vi "TimeGatedImage.vi"(2 "Image Path":refnum<vi>, 3 "notes 3":refnum<vi>) -> ()   [LabVIEW 2009]
panel:
  in  "ADC-factor":u16
  out "Decays":u32[][](graph)
  in  "RGB / False":enum16{"RGB", "False color"}(ring)
  in  "router channel":u16
  in  "threshold":cluster{"max":u32, "min":u32}
  out "Counts":u32[](array[numeric])
  in  "Export":bool
  in  "notes":string
  in  "update":bool
  in  "return":bool
  # "S"
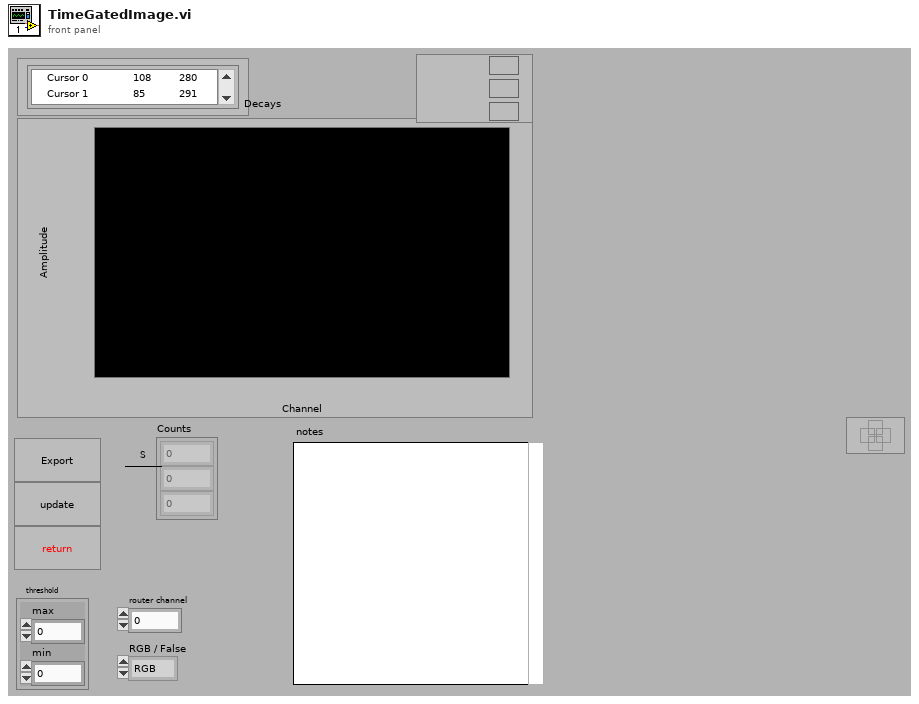
[diagram p1: front panel]
types:
  T1 = enum16{"Display", "change", "Get", "Set", "Set Ken"}
  T2 = enum16{"Ini", "Get", "Set", "Refresh", "dump", "move", "name"}
  T3 = typedef "FIFOSettings_BH.ctt" = cluster{"Measurement":cluster{"Binning (ms)":sgl, "External Trigger Condition":u16, "Stop Condition:":u16, "Stop Count":dbl, "Buffer Size (Photons)":u16, "No of Channels":u16, "Ext Latch Delay":i16}, "ADC":cluster{"Module":u16, "ADC Resolution":i32, "Dither Range":i16, "Count Increment":i16, "Macro Time Clock":i16}, "SYNC":cluster{"SYNC ZC Level (mV)":sgl, "SYNC Freq Divider":i16, "SYNC Holdoff (ns)":sgl, "SYNC Threshold (mV)":sgl}, "TAC":cluster{"TAC Range (ns)":sgl, "TAC Gain":i16, "TAC Offset (%)":sgl, "TAC Limit Low (%)":sgl, "TAC Limit High (%)":sgl}, "CFD":cluster{"CFD Limit Low (mV)":sgl, "CFD Limit High (mV)":sgl, "CFD ZC Level (mV)":sgl, "CFD Holdoff (ns)":sgl}}
  T4 = typedef "Settings.ctl" = cluster{"threshold":cluster{"max":u32, "min":u32}, "RGB or false color":bool, "16bit":bool, "log/lin axis":u16, "spotsize button":bool, "Pixelsize":u16, "autoscale x":bool, "autoscale y":bool, "correlation":bool, "ADC-Resolution":i32, "F2-lifetime":cluster{"display tau":bool, "display F2":bool, "Palette Number lifetime":enum32{"Gray", "Binary", "Gradient", "Rainbow", "Temperature"}, "Palette Number F2":enum32{"Gray", "Binary", "Gradient", "Rainbow", "Temperature"}, "max tau-Value":dbl, "min tau-Value":dbl, "max F2-Value":dbl, "min F2-Value":dbl}, "TAC-Window 1":u16, "TAC-Window 2":u16, "false color palette":cluster{"1":u32, "2":u32, "3":u32, "4":u32, "5":u32, "6":u32, "7":u32, "8":u32, "8 2":u32, "8 3":u32, "8 4":u32, "8 5":u32}}
  T5 = typedef "ImageSettings.ctt" = cluster{"Start Position (µm)":cluster{"x":dbl, "y":dbl, "z":dbl}, "End Position (µm)":cluster{"x":dbl, "y":dbl, "z":dbl}, "Image Resolution (nm/pixel)":cluster{"x":dbl, "y":dbl, "z":dbl}, "Image Size (µm)":cluster{"x":dbl, "y":dbl, "z":dbl}, "Image Size (pixel)":cluster{"x":u32, "y":u32, "z":u32}, "Time Resolution\n(ms/pixel)":dbl, "1st Axis":u16, "2nd Axis":u16, "Retrace":bool, "Estimated Time":string}
  T6 = cluster{"router":u8[], "macro times":dbl[], "micro times":u16[], "invalid":dbl[], "gap":dbl[]}
  T7 = typedef "IMAQ Image.ctl" = refnum<image>
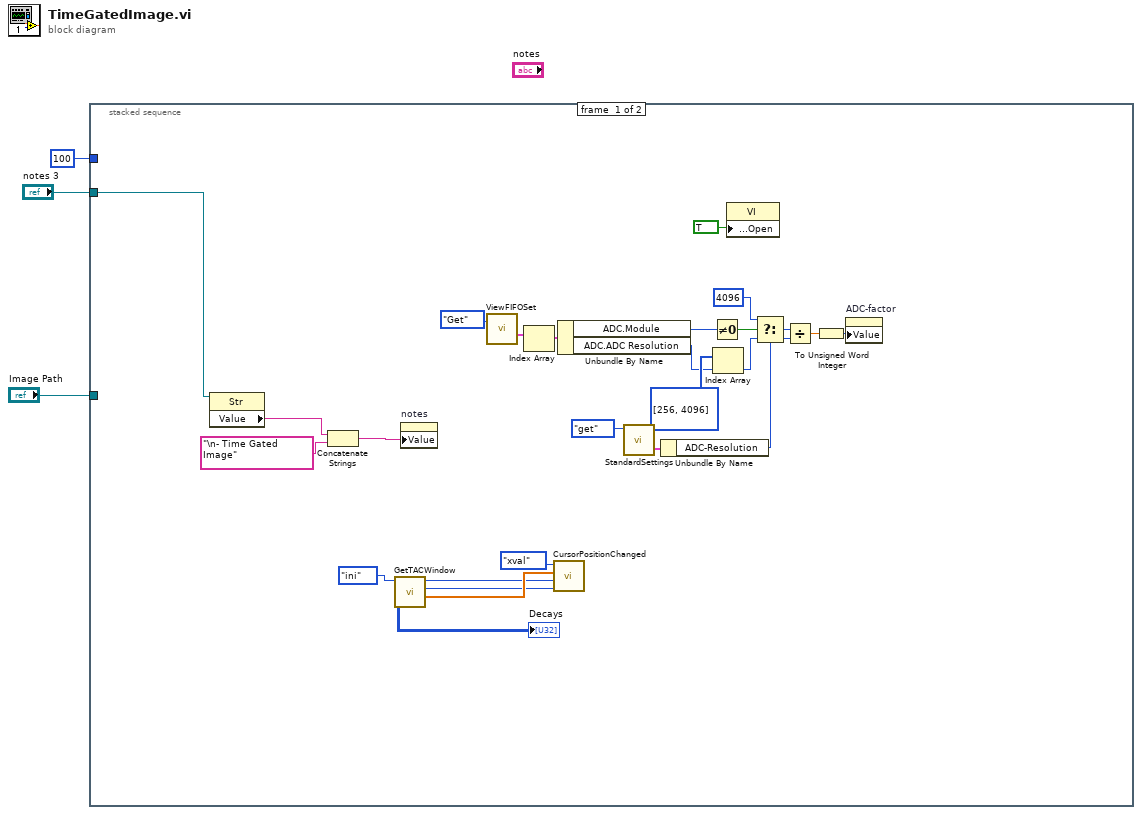
[diagram p0: block diagram]
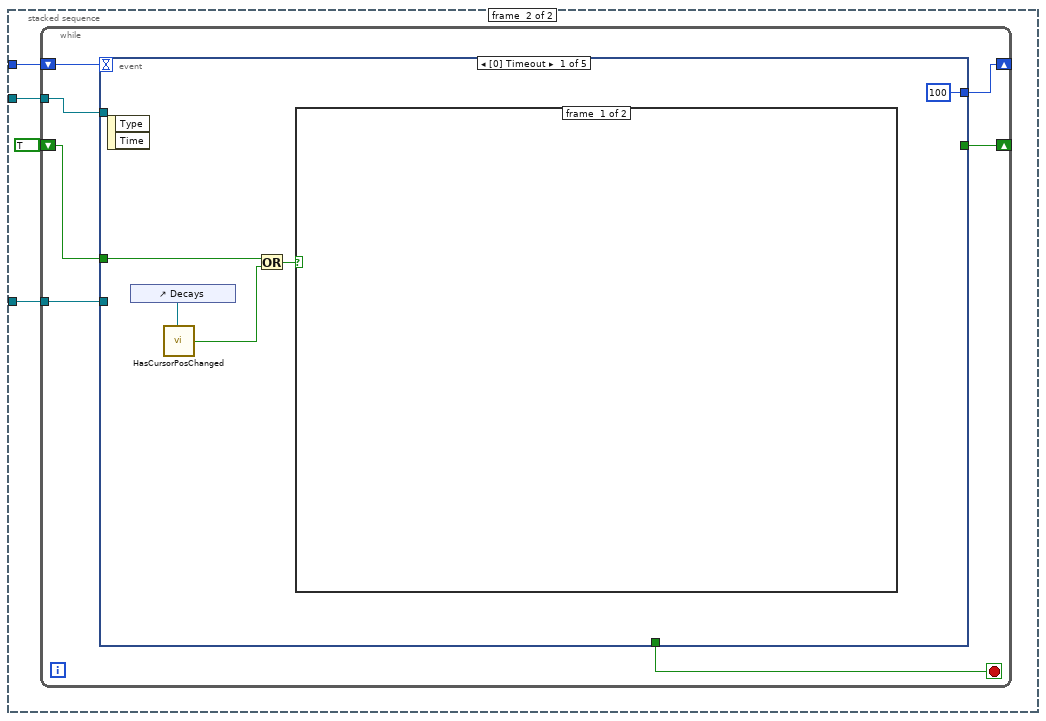
[diagram p2: hidden frame]
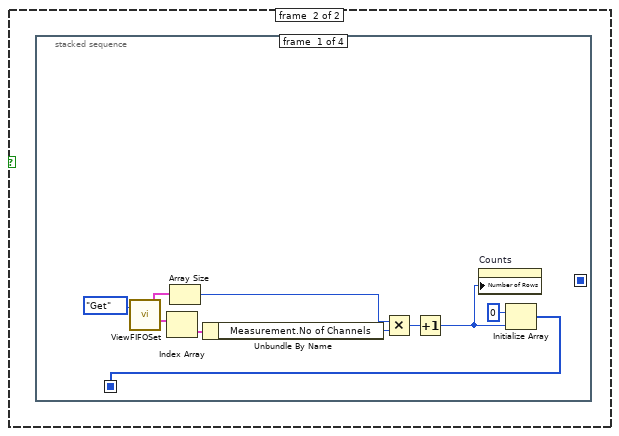
[diagram p3: hidden frame]
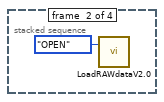
[diagram p4: hidden frame]
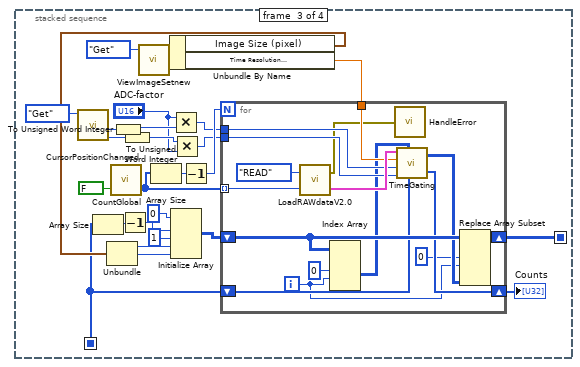
[diagram p5: hidden frame]
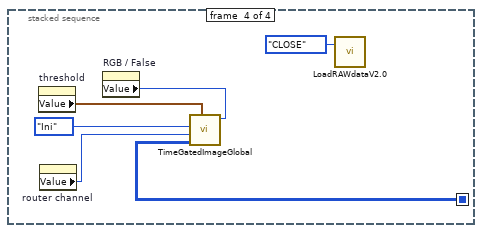
[diagram p6: hidden frame]
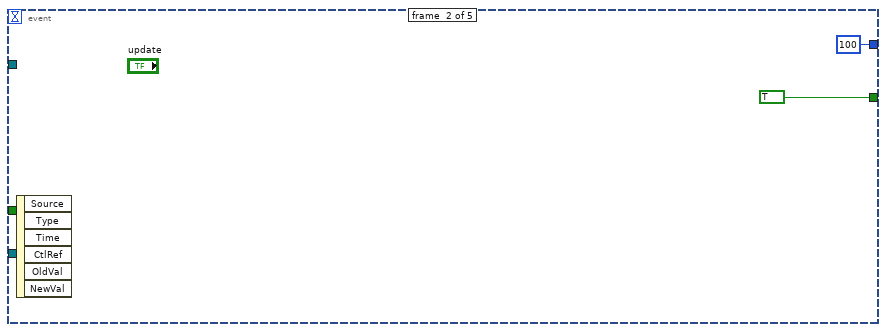
[diagram p7: hidden frame]
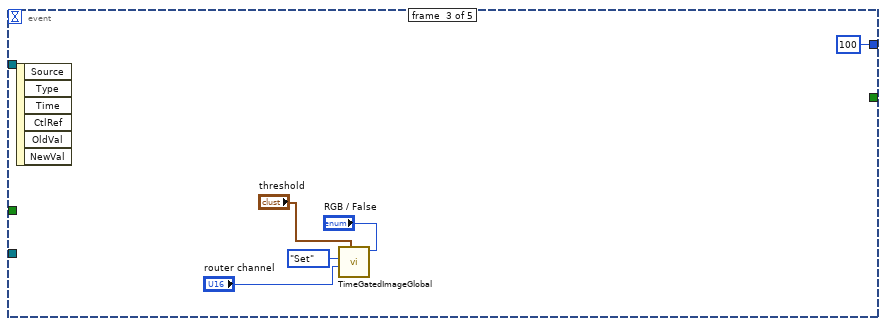
[diagram p8: hidden frame]
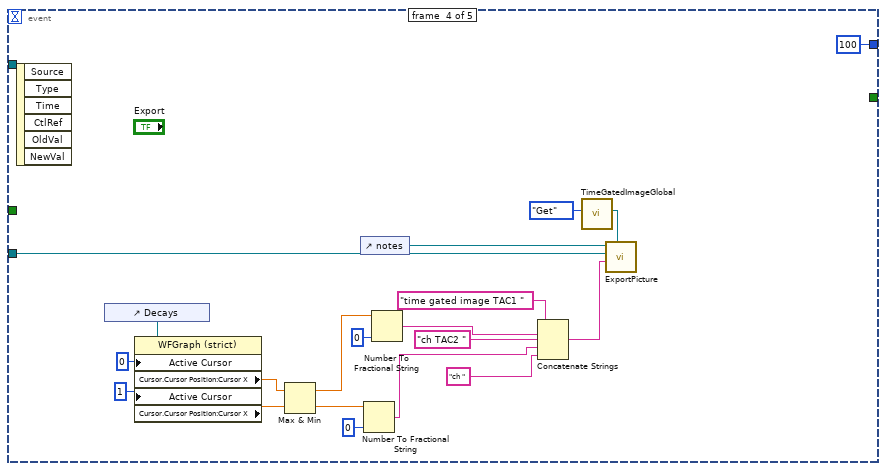
[diagram p9: hidden frame]
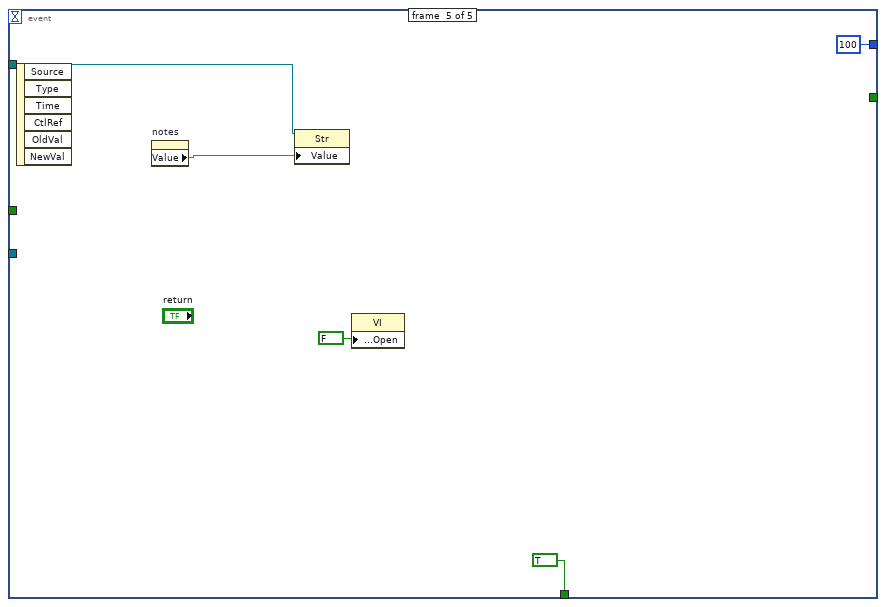
[diagram p10: hidden frame]
diagram:
  n1 = stacked-sequence {
    tunnel: "notes 3" -> [w19 w32]
    tunnel: 100 -> [_ w33]
    tunnel: "Image Path" -> [_ w30]
    frame #0 {
      n2 = property class="Str"(reference=w19) -> ("Value"=w28:string)  [unwired: 1 in, 2 out]
      n3 = Concatenate Strings(w28, "\n- Time Gated Image" ("string")) -> (w27:string)
      n4 = call "GetTACWindow.vi"("Enum"=enum16{"ini", "get", "quick"}."ini") -> ("Decays"=→"Decays":u32[][], "Cursor.Cursor Position:Cursor X"=w22:u16, "Cursor.Cursor Position:Cursor X 2"=w21:u16, "x-values"=w24:dbl[])  [unwired: 1 in, 5 out]
      n5 = property on="notes" class="String"("Value"=w27) -> ()  [unwired: 2 in, 2 out]
      n6 = call "ViewFIFOSet.vi"("Enum"=T1."Get") -> ("FIFO Settings (Array)"=w15:T3[])  [unwired: 1 in]
      n7 = Index Array(array=w15) -> (element=w14:T3)  [unwired: 1 in]
      n8 = call "CursorPositionChanged.vi"("CursorPos x1"=w21, "CursorPos x0"=w22, "x-values"=w24, "action"=enum16{"Check", "Get", "xval"}."xval" ("Enum")) -> ()  [unwired: 4 out]
      n9 = Unbundle By Name(w14) -> ("ADC.Module"=w13:u16, "ADC.ADC Resolution"=w8:i32)
      n10 = call "StandardSettings.vi"("Enum"=enum16{"Load", "get", "Save", "set"}."get") -> ("StandardSettings"=w17:T4)  [unwired: 4 in]
      n11 = Unbundle By Name(w17) -> ("ADC-Resolution"=w6:i32)
      n12 = Not Equal To 0?(x=w13) -> (x != 0?=w12:bool)
      n13 = Index Array(array=i32[] [256, 4096], index=w8) -> (element=w9:i32)
      n14 = property class="VI"("Front Panel Window:Open"=TRUE) -> ()  [unwired: 2 in, 2 out]
      n15 = Select(t=4096 ("ADC-Resolution"), s=w12, f=w9) -> (s? t:f=w7:i32)
      n16 = Divide(x=w7, y=w6) -> (x/y=w5:dbl)
      n17 = To Unsigned Word Integer(number=w5) -> (unsigned 16bit integer=w4:u16)
      n18 = property on="ADC-factor" class="DigNum (strict)"("Value"=w4) -> ()  [unwired: 2 in, 2 out]
    }
    frame #1 {
      n19 = while {
        shift-right: [w38] -> _
        shift-left: w33 -> [w39]
        tunnel: w32 -> [w37]
        shift-right: [w36] -> _
        shift-left: TRUE ("update") -> [w35]
        tunnel: w30 -> [w34]
        stop <- w40 stop-if-true
        n20 = event shown="[0] Timeout" {
          selector: _ -> [_ _ _ _ _]
          dyn-events: _ -> [_ _ _ _ _]
          timeout: w39 -> [_ _ _ _ _]
          tunnel: [_ _ _ _ TRUE] -> w40
          tunnel: [100 100 100 100 100] -> w38
          tunnel: w37 -> [_ _ _ _ w132]
          tunnel: [_ TRUE ("update") _ _ _] -> w36
          tunnel: w35 -> [w41 _ _ _ _]
          tunnel: w34 -> [_ _ _ w127 _]
          event #0 {
            n21 = event-data() -> ()  [unwired: 1 in, 2 out]
            n22 = control-ref of="Decays"() -> (w44:refnum<vi>)
            n23 = call "HasCursorPosChanged.vi"("Decay reference"=w44) -> ("changed?"=w42:bool)
            n24 = Or(x=w41, y=w42) -> (x .or. y?=w43:bool)
            n25 = case shown="True" w43 {
              frame #0 {
              }
              frame #1 {
                n26 = stacked-sequence {
                  seq-local: [w48 _ _ _] -> [_ _ w67 _]
                  seq-local: [_ _ w62 _] -> [_ _ _ w102]
                  frame #0 {
                    n27 = call "ViewFIFOSet.vi"("Enum"=T1."Get") -> ("FIFO Settings (Array)"=w53:T3[])  [unwired: 1 in]
                    n28 = Index Array(array=w53) -> (element=w52:T3)  [unwired: 1 in]
                    n29 = Array Size(array=w53) -> (size(s)=w50:i32)
                    n30 = Unbundle By Name(w52) -> ("Measurement.No of Channels"=w51:u16)
                    n31 = Multiply(x=w50, y=w51) -> (x*y=w47:i32)
                    n32 = Increment(x=w47) -> (x+1=w46:i32)
                    n33 = property on="Counts" class="Arr (strict)"("Number of Rows"=w46) -> ()  [unwired: 2 in, 2 out]
                    n34 = Initialize Array(u32 0 ("element"), w46) -> (w48:u32[])
                  }
                  frame #1 {
                    n35 = call "LoadRAWdataV2.0.vi"("action"=enum16{"OPEN", "READ", "CLOSE", "DATASREENER"}."OPEN") -> ()  [unwired: 1 in, 2 out]
                  }
                  frame #2 {
                    n36 = call "CursorPositionChanged.vi"("action"=enum16{"Check", "Get", "xval"}."Get" ("Enum")) -> ("CursorPos min out"=w78:u16, "CursorPos max out"=w79:u16)  [unwired: 3 in, 2 out]
                    n37 = Array Size(array=w67) -> (size(s)=w59:i32)
                    n38 = call "CountGlobal.vi"("changed?"=FALSE) -> ("count out"=w70:i32[])  [unwired: 2 in]
                    n39 = To Unsigned Word Integer(number=w79) -> (unsigned 16bit integer=w66:u16)
                    n40 = Decrement(x=w59) -> (x-1=w57:i32)
                    n41 = To Unsigned Word Integer(number=w78) -> (unsigned 16bit integer=w65:u16)
                    n42 = call "ViewImageSetnew.vi"("action"=T1."Get" ("Enum")) -> ("Image Settings"=w75:T5)  [unwired: 2 in]
                    n43 = Array Size(array=w70) -> (size(s)=w69:i32)
                    n44 = Unbundle By Name(w75) -> ("Image Size (pixel)"=w72:cluster{"x":u32, "y":u32, "z":u32}, "Time Resolution\n(ms/pixel)"=w74:dbl)
                    n45 = Unbundle(w72) -> ("x"=w60:u32, "y"=w61:u32)  [unwired: 1 out]
                    n46 = Multiply(x="ADC-factor", y=w66) -> (x*y=w63:u16)
                    n47 = Initialize Array(u32 0 ("element"), w57, u32 1 ("element"), w60, w61) -> (w73:u32[][][][])
                    n48 = Multiply(x=w65, y="ADC-factor") -> (x*y=w64:u16)
                    n49 = Decrement(x=w69) -> (x-1=w68:i32)
                    n50 = for {
                      N: w68 -> [_]
                      tunnel: w70 -> [w97] mode=indexing
                      tunnel: w63 -> [w91]
                      tunnel: w64 -> [w92]
                      tunnel: w74 -> [w90]
                      shift-right: [w94] -> w62
                      shift-left: w73 -> [w95]
                      shift-right: [w86] -> w71
                      shift-left: w67 -> [w87]
                      i -> [w82]
                      n51 = call "LoadRAWdataV2.0.vi"("pos offset (0)"=w97, "action"=enum16{"OPEN", "READ", "CLOSE", "DATASREENER"}."READ") -> ("RAW data"=w93:T6, "error out"=w85:errorcluster)
                      n52 = Index Array(array=w95, index (dim 1)=0 ("disabled index (page)"), index (dim 2)=w82) -> (element=w89:u32[][])  [unwired: 2 in]
                      n53 = call "HandleError.vi"("error in (no error)"=w85) -> ()
                      n54 = call "TimeGating.vi"("Counts"=w87, "Line Intensity in"=w89, "CursorPos min out"=w92, "CursorPos max out"=w91, "Time Resolution\n(ms/pixel)"=w90, "RAW data"=w93) -> ("Counts out"=w86:u32[], "Line Intensity out"=w88:u32[][])
                      n55 = Replace Array Subset(array=w95, new element=w88, index (dim 1)=0 ("disabled index (page)"), index (dim 2)=w82) -> (w94:u32[][][][])  [unwired: 2 in]
                    }
                    "Counts" <- w71
                  }
                  frame #3 {
                    n56 = property on="threshold" class="Cluster (strict)"() -> ("Value"=w100:cluster{"max":u32, "min":u32})  [unwired: 2 in, 2 out]
                    n57 = property on="router channel" class="DigNum (strict)"() -> ("Value"=w99:u16)  [unwired: 2 in, 2 out]
                    n58 = property on="RGB / False" class="Enum (strict)"() -> ("Value"=w98:enum16{"RGB", "False color"})  [unwired: 2 in, 2 out]
                    n59 = call "TimeGatedImageGlobal.vi"("RGB / False"=w98, "threshold"=w100, "input"=w102, "router channel"=w99, "action"=T2."Ini") -> ()  [unwired: 3 in, 2 out]
                    n60 = call "LoadRAWdataV2.0.vi"("action"=enum16{"OPEN", "READ", "CLOSE", "DATASREENER"}."CLOSE") -> ()  [unwired: 1 in, 2 out]
                  }
                }
              }
            }
          }
          event #1 {
            n61 = event-data() -> ()  [unwired: 1 in, 6 out]
          }
          event #2 {
            n62 = event-data() -> ()  [unwired: 1 in, 6 out]
            n63 = call "TimeGatedImageGlobal.vi"("RGB / False"="RGB / False", "threshold"="threshold", "router channel"="router channel", "action"=T2."Set") -> ()  [unwired: 4 in, 2 out]
          }
          event #3 {
            n64 = event-data() -> ()  [unwired: 1 in, 6 out]
            n65 = control-ref of="Decays"() -> (w125:refnum<vi>)
            n66 = property class="WFGraph (strict)"(reference=w125, "Active Cursor"=u32 0, "Active Cursor"=u32 1) -> ("Cursor.Cursor Position:Cursor X"=w111:dbl, "Cursor.Cursor Position:Cursor X"=w122:dbl)  [unwired: 1 in, 2 out]
            n67 = Max & Min(x=w111, y=w122) -> (max(x,y)=w113:dbl, min(x,y)=w112:dbl)
            n68 = control-ref of="notes"() -> (w126:refnum<vi>)
            n69 = Number To Fractional String(number=w112, precision (6)=i16 0) -> (F-format string=w116:string)  [unwired: 2 in]
            n70 = Number To Fractional String(number=w113, precision (6)=i16 0) -> (F-format string=w117:string)  [unwired: 2 in]
            n71 = Concatenate Strings("time gated image TAC1 ", w117, "ch TAC2 ", w116, "ch ") -> (w115:string)
            n72 = call "TimeGatedImageGlobal.vi"("action"=T2."Get") -> ("Image Duplicate (out)"=w128:T7)  [unwired: 7 in, 1 out]
            n73 = call "ExportPicture.vi"("Image"=w128, "name input"=w115, "Path"=w127, "notes 2"=w126) -> ()  [unwired: 3 in, 2 out]
          }
          event #4 {
            n74 = event-data() -> ()  [unwired: 1 in, 6 out]
            n75 = property on="notes" class="String"() -> ("Value"=w131:string)  [unwired: 2 in, 2 out]
            n76 = property class="Str"(reference=w132, "Value"=w131) -> ()  [unwired: 1 in, 2 out]
            n77 = property class="VI"("Front Panel Window:Open"=FALSE) -> ()  [unwired: 2 in, 2 out]
          }
        }
      }
    }
  }
